vi "Main3.vi"() -> ()   [LabVIEW 2014]
uses:
  Enum State Typedef.ctl
  <vilib>/Utility/error.llb/DialogType.ctl
  <vilib>/_DAQmxBase/Internals/DAQmxBase Create Channel (AI-Voltage-Basic).vi
  <vilib>/_DAQmxBase/Internals/DAQmxBase Timing (Sample Clock).vi
  <vilib>/_DAQmxBase/Internals/DAQmxBase Read (Analog 2D DBL NChan NSamp).vi
  <vilib>/Utility/file.llb/Write To Spreadsheet File (DBL).vi
panel:
  in  "OK Button":bool
  in  "Physical channel":tag
  out "State":T1
  in  "Clear Display":bool
  in  "Preview Button":bool
  out "size(s)":i32
  in  "pH":dbl
  in  "Conductivity (mS)":dbl
  out "Iterations Recorded":i32
  in  "Recording Time (seconds)":dbl
  in  "Sample Rate":i32=1000
  in  "Stop Button":bool
  out "Waveform Chart":waveform(dbl)(graph)
  in  "High Pass Filter":enum16{"500", "1k", "5k", "10k", "20k"}(ring)
  in  "Low Pass Filter":enum16{"0.1", "1.0", "10", "100", "300"}(ring)
  in  "Gain":enum16{"x100", "x1000", "x10k"}(ring)
  in  "Notch Filter":bool
  in  "Amplifier Model":u16(ring) items=["Select a Model", "AM 1700", "BMA 200"]
  in  "AC/DC Switch":bool
  in  "Temperature (deg C)":dbl
  in  "User Comments":string
  out "Start Time hr/min":string
  out "Date mm/dd/yy":string
  in  "Species":string
  in  "Exit Button":bool
  in  "Record Button":bool
  # "MSU EFISH Lab Single Channel Electronic Pulse Recorder"
  # "Must enter numbers into here before you start"
  # "Blue for On\nOrange for Off"
  # "DC"
  # "AC"
  # "Blue for AC and Orange for DC"
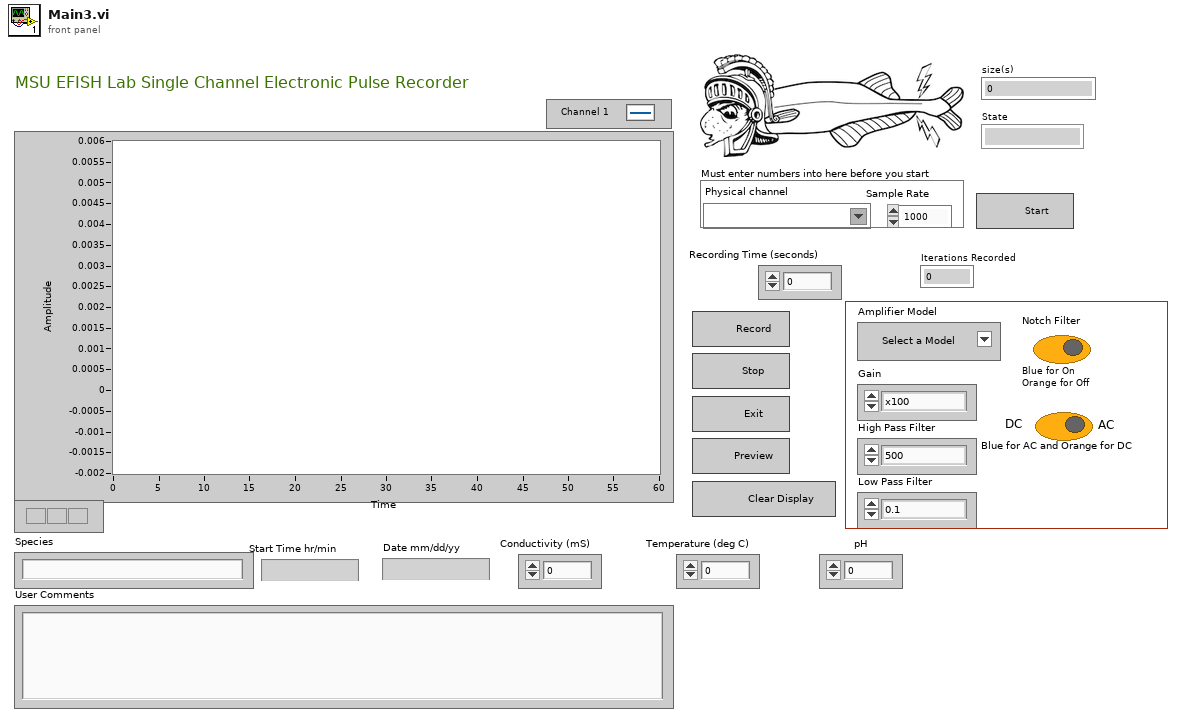
[diagram p1: front panel]
types:
  T1 = typedef "Enum State Typedef.ctl" = enum16{"", "Beginning State", "Set the Sample Clock", "Prepreview Handling", "Clear Display", "Preview Data", "Stop", "Exit", "Record", "Create File"}
  T2 = typedef "DialogType.ctl" = u16
  T3 = cluster{"High Pass Filter":enum16{"500", "1k", "5k", "10k", "20k"}, "Gain":enum16{"x100", "x1000", "x10k"}, "Low Pass Filter":enum16{"0.1", "1.0", "10", "100", "300"}, "Amplifier Model":u16, "Notch Filter":bool, "AC/DC Switch":bool, "Temperature (deg C)":dbl, "Conductivity (mS)":dbl, "pH":dbl, "User Comments":string, "Species":string}
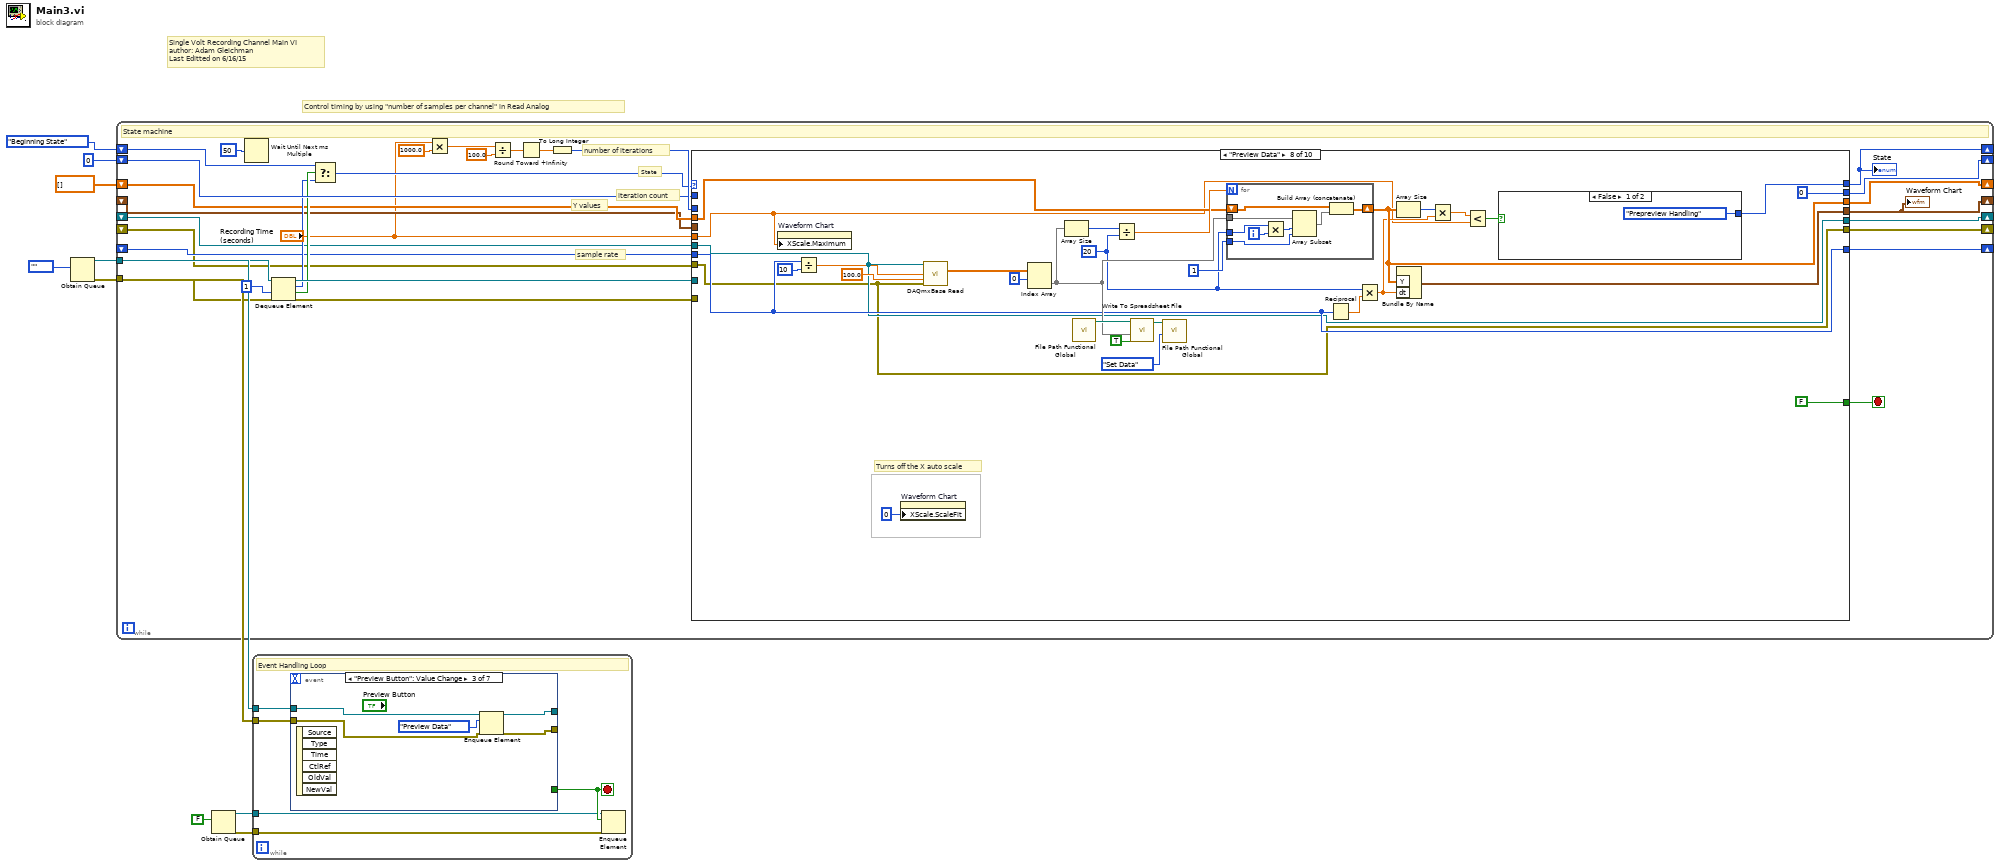
[diagram p0: block diagram]
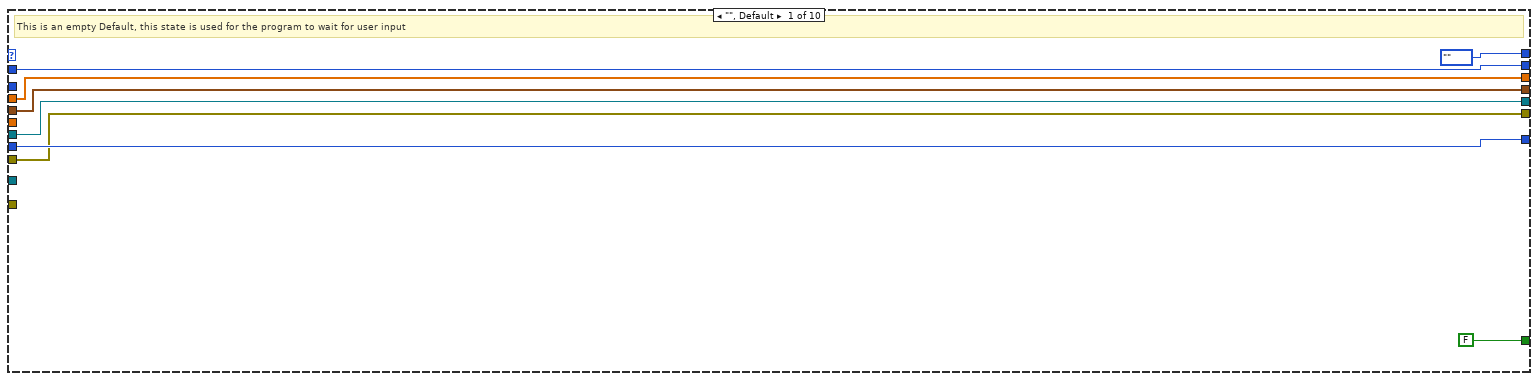
[diagram p2: hidden frame]
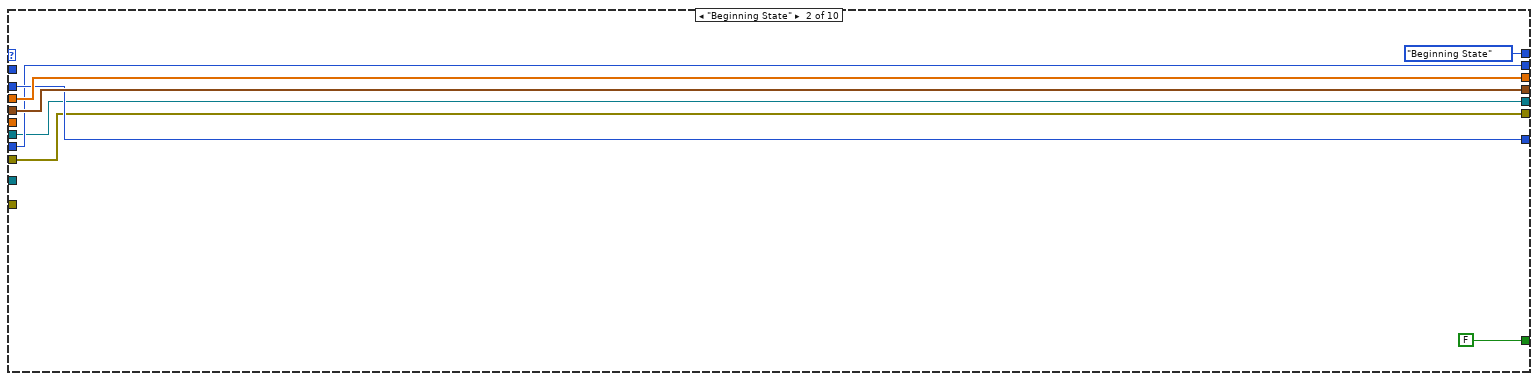
[diagram p3: hidden frame]
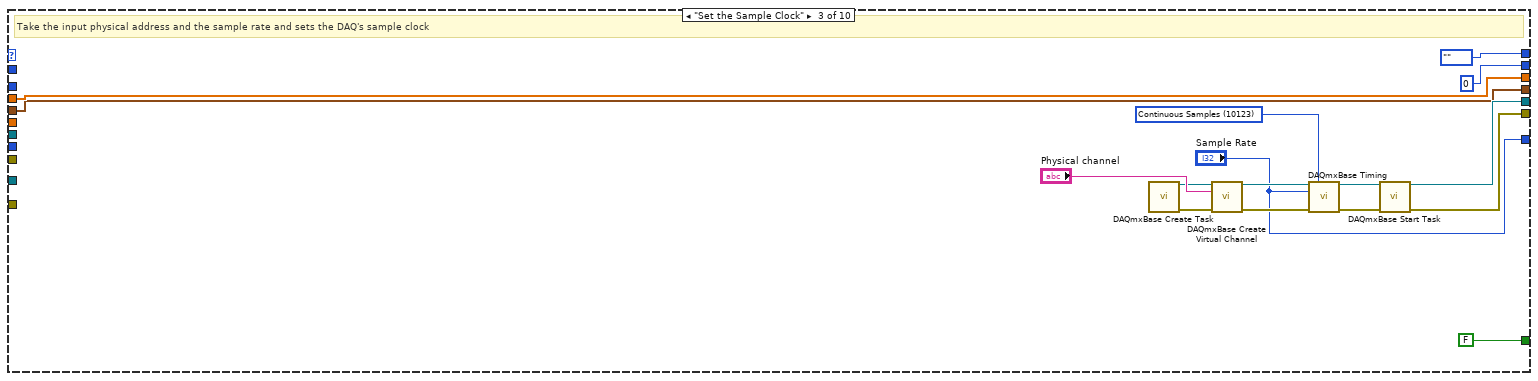
[diagram p4: hidden frame]
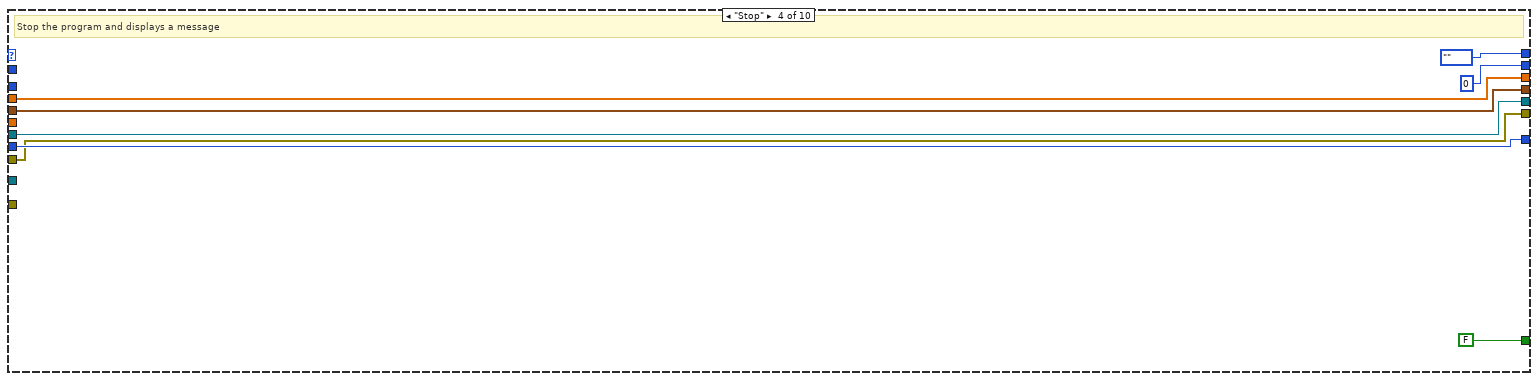
[diagram p5: hidden frame]
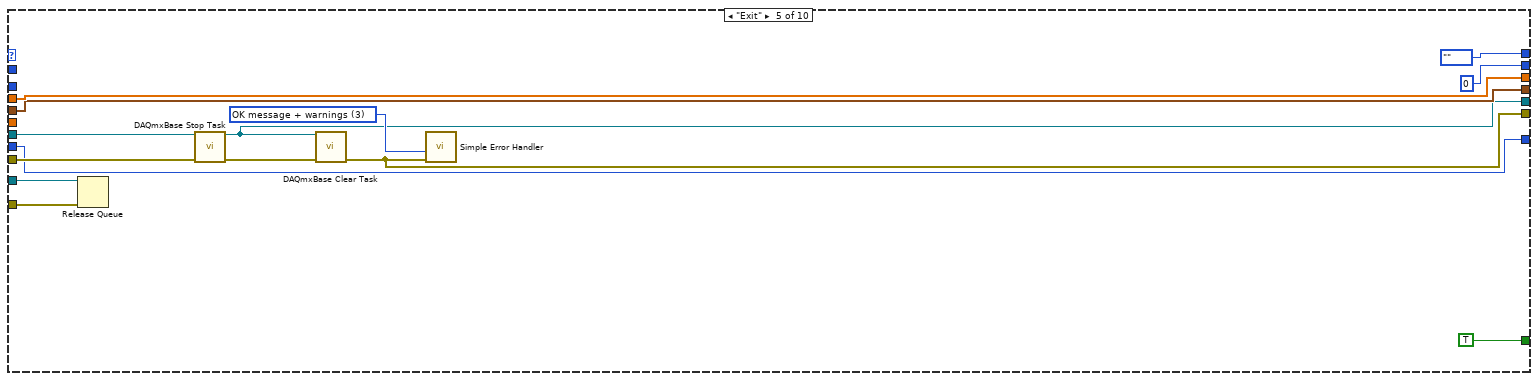
[diagram p6: hidden frame]
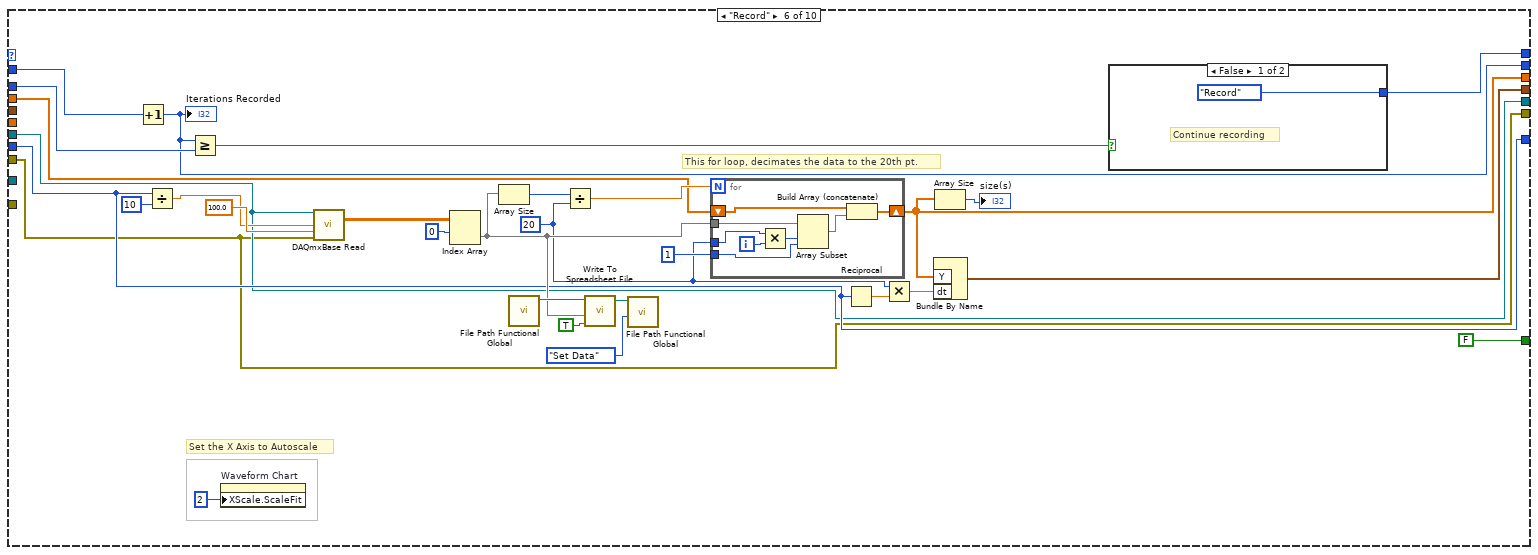
[diagram p7: hidden frame]
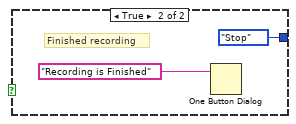
[diagram p8: hidden frame]
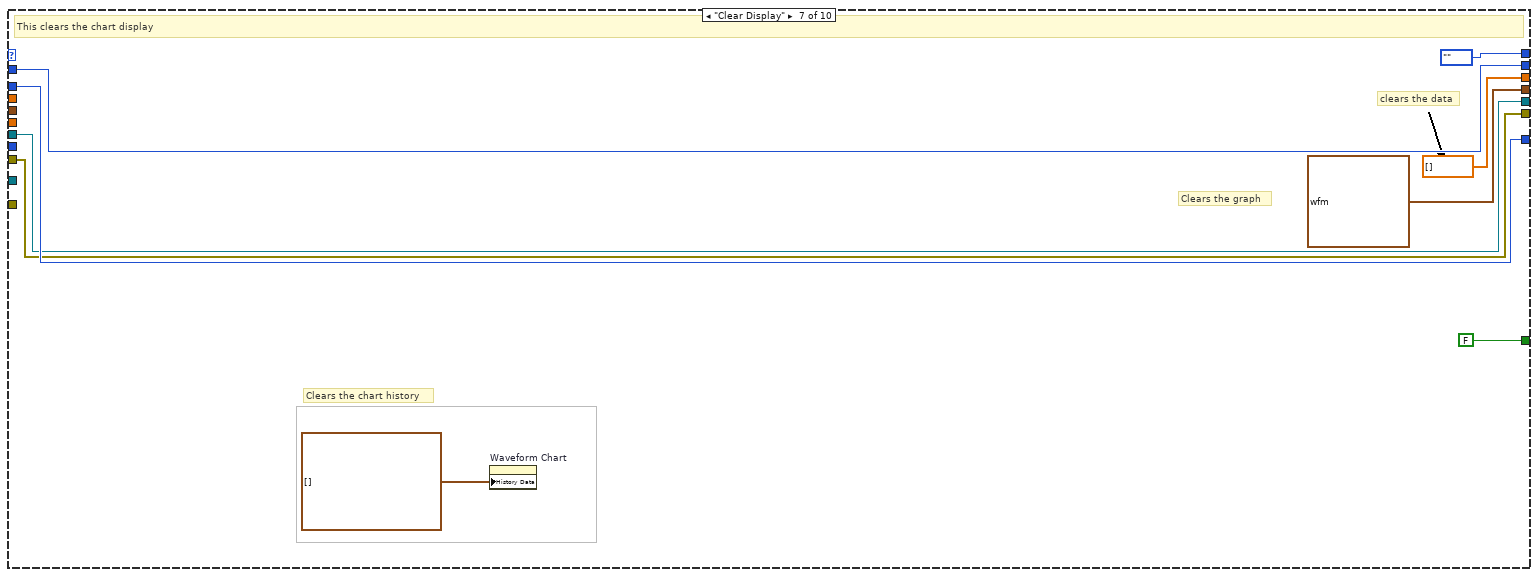
[diagram p9: hidden frame]
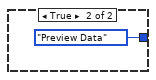
[diagram p10: hidden frame]
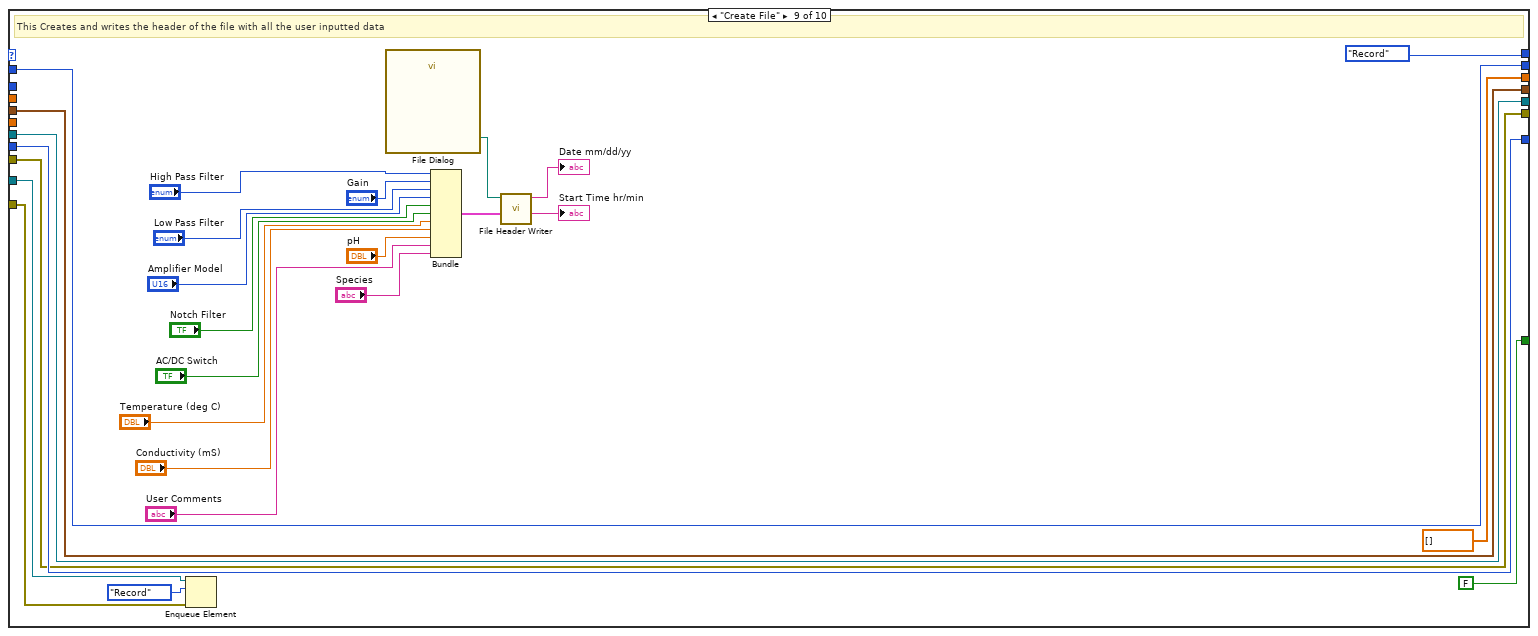
[diagram p11: hidden frame]
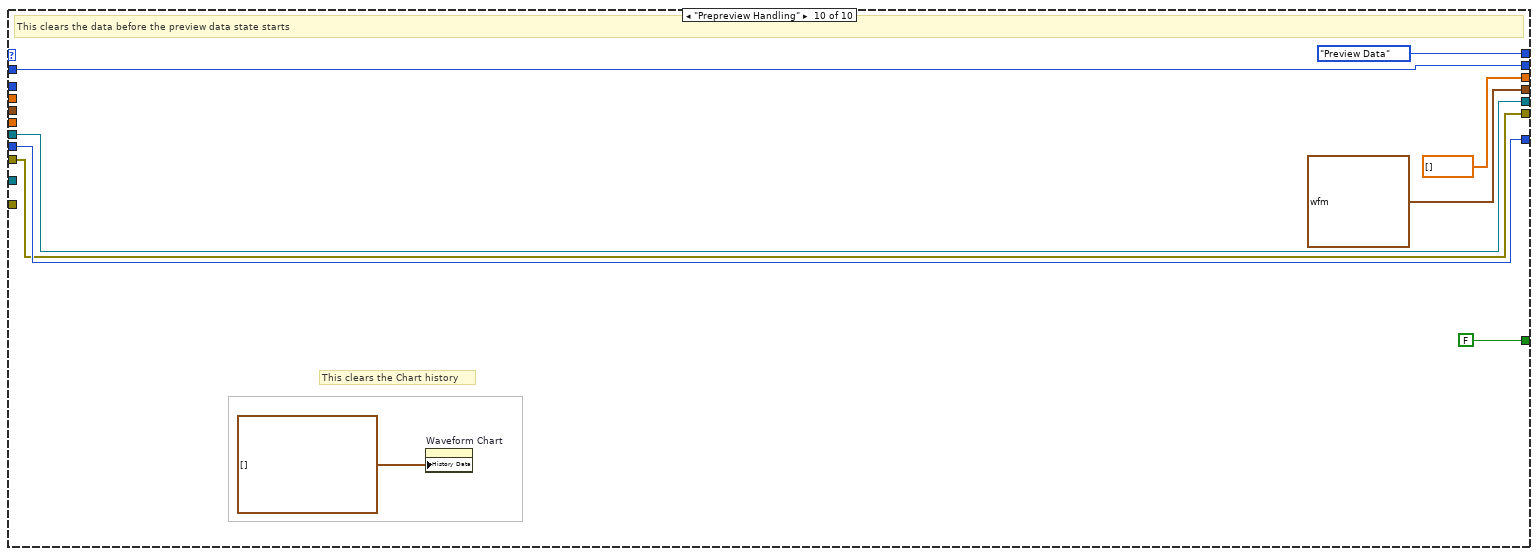
[diagram p12: hidden frame]
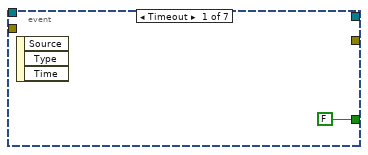
[diagram p13: hidden frame]
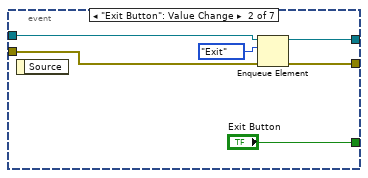
[diagram p14: hidden frame]
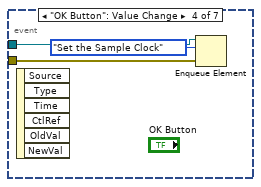
[diagram p15: hidden frame]
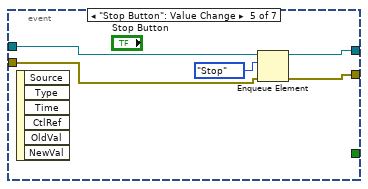
[diagram p16: hidden frame]
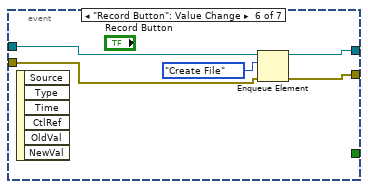
[diagram p17: hidden frame]
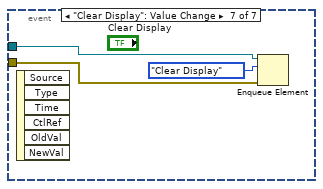
[diagram p18: hidden frame]
diagram:
  # "Single Volt Recording Channel Main VI\nauthor: Adam Gleichman\nLast Editted on 6/16/15"
  # "Control timing by using \"number of samples per channel\" in Read Analog"
  n1 = Obtain Queue(element data type=Enum_State_Typedef."" ("State")) -> (queue out=w8:refnum<queue>, error out=w7:errorcluster)  [unwired: 4 in, 1 out]
  n2 = while {
    tunnel: w8 -> [w40]
    tunnel: w7 -> [w39]
    shift-right: [w28] -> _
    shift-left: 0 -> [w29]
    shift-right: [w23] -> _
    shift-left: Enum_State_Typedef."Beginning State" ("State") -> [w25]
    shift-right: [w21] -> _
    shift-left: _ -> [w22]
    shift-right: [w15] -> _
    shift-left: dbl[] [] -> [w18]
    shift-right: [w17] -> _
    shift-left: _ -> [w16]
    shift-right: [w13] -> _
    shift-left: _ -> [w11]
    shift-right: [w12] -> _
    shift-left: _ -> [w10]
    stop <- w38 stop-if-true
    # "State"
    # "iteration count"
    # "Y values"
    # "sample rate"
    # "number of iterations"
    # "State machine"
    n3 = Wait Until Next ms Multiple(millisecond multiple=u32 50) -> ()  [unwired: 1 out]
    n4 = Dequeue Element(queue=w40, timeout in ms (-1)=1, error in (no error)=w39) -> (queue out=w37:refnum<queue>, element=w26:T1, timed out?=w27:bool, error out=w36:errorcluster)
    n5 = Select(t=w25, s=w27, f=w26) -> (s? t:f=w24:T1)
    n6 = Multiply(x="Recording Time (seconds)", y=1000.0) -> (x*y=w34:dbl)
    n7 = Divide(x=w34, y=100.0) -> (x/y=w32:dbl)
    n8 = Round Toward +Infinity(x=w32) -> (ceil(x): smallest int >= x=w31:dbl)
    n9 = To Long Integer(number=w31) -> (32bit integer=w30:i32)
    n10 = case shown="\"Preview Data\"" w24 {
      tunnel: [FALSE FALSE FALSE FALSE TRUE FALSE FALSE FALSE FALSE FALSE] -> w38
      tunnel: w37 -> [_ _ _ _ w89 _ _ _ w210 _]
      tunnel: w36 -> [_ _ _ _ w88 _ _ _ w209 _]
      tunnel: w11 -> [w42 w50 _ w74 w92 w96 w137 w146 w186 w212]
      tunnel: w10 -> [w41 w51 _ w73 w91 w95 w136 w145 w185 w211]
      tunnel: w22 -> [w45 w52 _ w77 w85 w101 _ w153 w206 w214]
      tunnel: w30 -> [_ w53 _ _ _ w117 w141 _ _ _]
      tunnel: w29 -> [w47 _ _ _ _ w118 w144 _ w207 w215]
      tunnel: [w47 w52 0 ("Sample Rate") 0 0 w112 w144 0 w207 w215] -> w28
      tunnel: [Enum_State_Typedef."" ("State") Enum_State_Typedef."Beginning State" ("State") Enum_State_Typedef."" ("State") Enum_State_Typedef."" ("State") Enum_State_Typedef."" ("State") w114 Enum_State_Typedef."" ("State") w155 Enum_State_Typedef."Record" ("State") Enum_State_Typedef."Preview Data" ("State")] -> w23
      tunnel: [w45 w53 "Sample Rate" w77 w85 w101 w141 w153 w206 w214] -> w21
      tunnel: [w44 w55 w61 w76 w84 w105 dbl[] [] w154 dbl[] [] dbl[] []] -> w15
      tunnel: w18 -> [w44 w55 w61 w76 w84 w104 _ w157 _ _]
      tunnel: [w43 w54 w60 w75 w83 w103 waveform(dbl) {"t0"=timestamp(0 s since 1904-01-01), "dt"=1.0, "Y"=[]} w156 w194 waveform(dbl) {"t0"=timestamp(0 s since 1904-01-01), "dt"=1.0, "Y"=[]}] -> w17
      tunnel: w16 -> [w43 w54 w60 w75 w83 _ _ _ w194 _]
      tunnel: "Recording Time (seconds)" -> [_ _ _ _ _ _ _ w148 _ _]
      tunnel: [w42 w50 w64 w74 w82 w96 w137 w146 w186 w212] -> w13
      tunnel: [w41 w51 w63 w73 w81 w95 w136 w145 w185 w211] -> w12
      frame "", Default {
        # "This is an empty Default, this state is used for the program to wait for user input"
      }
      frame "Beginning State" {
      }
      frame "Set the Sample Clock" {
        w67 = 10123 items=["Finite Samples"=10178, "Continuous Samples"=10123, "Hardware Timed Single Point"=12522] ("sample mode")
        # "Take the input physical address and the sample rate and sets the DAQ's sample clock"
        n11 = call <vilib>:"DAQmxBase Create Task.vi"() -> ("task out"=w71:refnum<k21>, "error out"=w70:errorcluster)  [unwired: 14 in]
        n12 = call-poly <vilib>:"DAQmxBase Create Virtual Channel.vi"("task in"=w71, "physical channels"="Physical channel", "error in"=w70) -> ("task out"=w69:refnum<k21>, "error out"=w68:errorcluster)  [unwired: 11 in]
        n13 = call-poly <vilib>:"DAQmxBase Timing.vi"("task/channels in"=w69, "sample mode"=w67, "rate"="Sample Rate", "error in"=w68) -> ("task out"=w66:refnum<k21>, "error out"=w65:errorcluster)  [unwired: 10 in]
        n14 = call <vilib>:"DAQmxBase Start Task.vi"("task/channels in"=w66, "error in"=w65) -> ("task out"=w64:refnum<k21>, "error out"=w63:errorcluster)  [unwired: 12 in]
      }
      frame "Stop" {
        # "Stop the program and displays a message"
      }
      frame "Exit" {
        w90 = T2 3 items=["no dialog", "OK message", "continue or stop message", "OK message + warnings", "continue/stop + warnings"] ("type of dialog (OK msg:1)")
        n15 = Release Queue(queue=w89, error in (no error)=w88) -> ()  [unwired: 1 in, 3 out]
        n16 = call <vilib>:"DAQmxBase Stop Task.vi"("task/channels in"=w92, "error in"=w91) -> ("task out"=w82:refnum<k21>, "error out"=w93:errorcluster)  [unwired: 12 in]
        n17 = call <vilib>:"DAQmxBase Clear Task.vi"("task in"=w82, "error in"=w93) -> ("error out"=w81:errorcluster)  [unwired: 13 in]
        n18 = call <vilib>:"Simple Error Handler.vi"("type of dialog (OK msg:1)"=w90, "error in (no error)"=w81) -> ()  [unwired: 3 in, 5 out]
      }
      frame "Record" {
        w99 = 20 ("y")
        # "This for loop, decimates the data to the 20th pt."
        # "Set the X Axis to Autoscale"
        n19 = Increment(x=w118) -> (x+1=w112:i32)
        "Iterations Recorded" <- w112
        n20 = Divide(x=w101, y=10) -> (x/y=w115:dbl)
        n21 = Greater Or Equal?(x=w112, y=w117) -> (x >= y?=w113:bool)
        n22 = property on="Waveform Chart" class="WFChart (strict)"("XScale.ScaleFit"=u8 2 ("X Scale.Scale Fit")) -> ()  [unwired: 2 in, 2 out]
        n23 = call-poly <vilib>:"DAQmxBase Read.vi"("task/channels in"=w96, "number of samples per channel"=w115, "timeout"=100.0, "error in"=w95) -> ("data"=w110:dbl[][])  [unwired: 9 in, 2 out]
        n24 = Index Array(array=w110, index (row)=0) -> (element=w102:dbl[])  [unwired: 1 in]
        n25 = Array Size(array=w102) -> (size(s)=w109:i32)
        n26 = call "File Path Functional Global.vi"() -> ("File Path Output"=w122:path)  [unwired: 11 in]
        n27 = Divide(x=w109, y=w99) -> (x/y=w108:dbl)
        n28 = call-poly <vilib>:"Write To Spreadsheet File.vi"("append to file? (new file:F)"=TRUE, "1D data"=w102, "file path (dialog if empty)"=w122) -> ("new file path (Not A Path if cancelled)"=w120:path)  [unwired: 5 in]
        n29 = call "File Path Functional Global.vi"("Enum"=enum16{"Get Data", "Set Data"}."Set Data", "File Path Control"=w120) -> ()  [unwired: 9 in, 1 out]
        n30 = for {
          N: w108 -> [_]
          shift-right: [w125] -> w105
          shift-left: w104 -> [w127]
          tunnel: w102 -> [w132]
          tunnel: w99 -> [w130]
          tunnel: 1 ("y") -> [w128]
          i -> [w131]
          n31 = Multiply(x=w130, y=w131) -> (x*y=w129:i32)
          n32 = Array Subset(array=w132, index=w129, length=w128) -> (w126:dbl[])
          n33 = Build Array (concatenate)(w127, w126) -> (w125:dbl[])
        }
        n34 = Reciprocal(x=w101) -> (1/x=w100:dbl)
        n35 = Multiply(x=w99, y=w100) -> (x*y=w98:dbl)
        n36 = Bundle By Name("Y"=w105, "dt"=w98) -> (w103:waveform(dbl))  [unwired: 1 in]
        n37 = Array Size(array=w105) -> (size(s)=→"size(s)":i32)
        n38 = case shown="False" w113 {
          tunnel: [Enum_State_Typedef."Record" ("State") Enum_State_Typedef."Stop" ("State")] -> w114
          frame False {
            # "Continue recording"
          }
          frame True {
            # "Finished recording"
            n39 = One Button Dialog(message="Recording is Finished") -> ()  [unwired: 1 in, 1 out]
          }
        }
      }
      frame "Clear Display" {
        # "clears the data"
        # "Clears the graph"
        # "Clears the chart history"
        # "This clears the chart display"
        n40 = property on="Waveform Chart" class="WFChart (strict)"("History Data"=waveform(dbl)[] []) -> ()  [unwired: 2 in, 2 out]
      }
      frame "Preview Data" {
        w158 = 20 ("y")
        # "Turns off the X auto scale"
        n41 = property on="Waveform Chart" class="WFChart (strict)"("XScale.Maximum"=w148) -> ()  [unwired: 2 in, 2 out]
        n42 = Divide(x=w153, y=10) -> (x/y=w166:dbl)
        n43 = property on="Waveform Chart" class="WFChart (strict)"("XScale.ScaleFit"=u8 0 ("X Scale.Scale Fit")) -> ()  [unwired: 2 in, 2 out]
        n44 = call-poly <vilib>:"DAQmxBase Read.vi"("task/channels in"=w146, "number of samples per channel"=w166, "timeout"=100.0, "error in"=w145) -> ("data"=w164:dbl[][])  [unwired: 9 in, 2 out]
        n45 = Index Array(array=w164, index (row)=0) -> (element=w160:dbl[])  [unwired: 1 in]
        n46 = Array Size(array=w160) -> (size(s)=w163:i32)
        n47 = call "File Path Functional Global.vi"() -> ("File Path Output"=w171:path)  [unwired: 11 in]
        n48 = Divide(x=w163, y=w158) -> (x/y=w162:dbl)
        n49 = call-poly <vilib>:"Write To Spreadsheet File.vi"("append to file? (new file:F)"=TRUE, "1D data"=w160, "file path (dialog if empty)"=w171) -> ("new file path (Not A Path if cancelled)"=w169:path)  [unwired: 5 in]
        n50 = call "File Path Functional Global.vi"("Enum"=enum16{"Get Data", "Set Data"}."Set Data", "File Path Control"=w169) -> ()  [unwired: 9 in, 1 out]
        n51 = for {
          N: w162 -> [_]
          shift-right: [w177] -> w154
          shift-left: w157 -> [w179]
          tunnel: w160 -> [w184]
          tunnel: w158 -> [w182]
          tunnel: 1 ("y") -> [w180]
          i -> [w183]
          n52 = Multiply(x=w182, y=w183) -> (x*y=w181:i32)
          n53 = Array Subset(array=w184, index=w181, length=w180) -> (w178:dbl[])
          n54 = Build Array (concatenate)(w179, w178) -> (w177:dbl[])
        }
        n55 = Reciprocal(x=w153) -> (1/x=w159:dbl)
        n56 = Multiply(x=w158, y=w159) -> (x*y=w150:dbl)
        n57 = Bundle By Name("Y"=w154, "dt"=w150) -> (w156:waveform(dbl))  [unwired: 1 in]
        n58 = Array Size(array=w154) -> (size(s)=w151:i32)
        n59 = Multiply(x=w151, y=w150) -> (x*y=w149:dbl)
        n60 = Less?(x=w149, y=w148) -> (x < y?=w152:bool)
        n61 = case shown="False" w152 {
          tunnel: [Enum_State_Typedef."Prepreview Handling" ("State") Enum_State_Typedef."Preview Data" ("State")] -> w155
          frame False {
          }
          frame True {
          }
        }
      }
      frame "Create File" {
        # "This Creates and writes the header of the file with all the user inputted data"
        n62 = Enqueue Element(queue=w210, element=Enum_State_Typedef."Record", error in (no error)=w209) -> ()  [unwired: 1 in, 3 out]
        n63 = call "File Dialog"() -> ("selected path"=w191:path)  [unwired: 12 in, 3 out]
        n64 = Bundle("High Pass Filter"="High Pass Filter", "Gain"="Gain", "Low Pass Filter"="Low Pass Filter", "Amplifier Model"="Amplifier Model", "Notch Filter"="Notch Filter", "AC/DC Switch"="AC/DC Switch", "Temperature (deg C)"="Temperature (deg C)", "Conductivity (mS)"="Conductivity (mS)", "pH"="pH", "User Comments"="User Comments", "Species"="Species") -> (w190:T3)  [unwired: 1 in]
        n65 = call "File Header Writer.vi"("Data Cluster"=w190, "File Path"=w191) -> ("Start Time hr/min"=→"Start Time hr/min":string, "Date mm/dd/yy"=→"Date mm/dd/yy":string)  [unwired: 8 in]
      }
      frame "Prepreview Handling" {
        # "This clears the Chart history"
        # "This clears the data before the preview data state starts"
        n66 = property on="Waveform Chart" class="WFChart (strict)"("History Data"=waveform(dbl)[] []) -> ()  [unwired: 2 in, 2 out]
      }
    }
    "Waveform Chart" <- w17
    "State" <- w23
  }
  n67 = Obtain Queue(element data type=FALSE) -> (queue out=w2:refnum<queue>, error out=w1:errorcluster)  [unwired: 4 in, 1 out]
  n68 = while {
    tunnel: w8 -> [w224]
    tunnel: w7 -> [w223]
    tunnel: w2 -> [w221]
    tunnel: w1 -> [w220]
    stop <- w222 stop-if-true
    # "Event Handling Loop"
    n69 = event shown="[2] \"Preview Button\": Value Change" {
      selector: _ -> [_ _ _ _ _ _ _]
      dyn-events: _ -> [_ _ _ _ _ _ _]
      timeout: _ -> [_ _ _ _ _ _ _]
      tunnel: [FALSE ("Exit Button") "Exit Button" _ _ _ _ _] -> w222
      tunnel: w224 -> [_ w230 w236 w239 w244 w249 w252]
      tunnel: w223 -> [_ w229 w235 w238 w243 w248 w251]
      tunnel: [_ w228 w233 _ w241 w246 _] -> _
      tunnel: [_ w227 w232 _ w242 w247 _] -> _
      event Timeout {
        n70 = event-data() -> ()  [unwired: 1 in, 3 out]
      }
      event "Exit Button": Value Change {
        n71 = event-data() -> ()  [unwired: 1 in, 1 out]
        n72 = Enqueue Element(queue=w230, element=Enum_State_Typedef."Exit", error in (no error)=w229) -> (queue out=w228:refnum<queue>, error out=w227:errorcluster)  [unwired: 1 in, 1 out]
      }
      event "Preview Button": Value Change {
        n73 = event-data() -> ()  [unwired: 1 in, 6 out]
        n74 = Enqueue Element(queue=w236, element=Enum_State_Typedef."Preview Data", error in (no error)=w235) -> (queue out=w233:refnum<queue>, error out=w232:errorcluster)  [unwired: 1 in, 1 out]
      }
      event "OK Button": Value Change {
        n75 = event-data() -> ()  [unwired: 1 in, 6 out]
        n76 = Enqueue Element(queue=w239, element=Enum_State_Typedef."Set the Sample Clock", error in (no error)=w238) -> ()  [unwired: 1 in, 3 out]
      }
      event "Stop Button": Value Change {
        n77 = event-data() -> ()  [unwired: 1 in, 6 out]
        n78 = Enqueue Element(queue=w244, element=Enum_State_Typedef."Stop", error in (no error)=w243) -> (queue out=w241:refnum<queue>, error out=w242:errorcluster)  [unwired: 1 in, 1 out]
      }
      event "Record Button": Value Change {
        n79 = event-data() -> ()  [unwired: 1 in, 6 out]
        n80 = Enqueue Element(queue=w249, element=Enum_State_Typedef."Create File", error in (no error)=w248) -> (queue out=w246:refnum<queue>, error out=w247:errorcluster)  [unwired: 1 in, 1 out]
      }
      event "Clear Display": Value Change {
        n81 = event-data() -> ()  [unwired: 1 in, 6 out]
        n82 = Enqueue Element(queue=w252, element=Enum_State_Typedef."Clear Display", error in (no error)=w251) -> ()  [unwired: 1 in, 3 out]
      }
    }
    n83 = Enqueue Element(queue=w221, element=w222, error in (no error)=w220) -> ()  [unwired: 1 in, 3 out]
  }
